vi "Lever.vi"(1 "Input":bool) -> (0 "Output":bool)   [LabVIEW 2017]
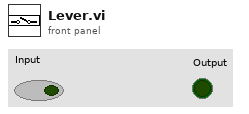
[diagram p1: front panel]
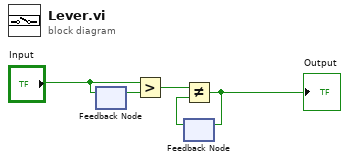
[diagram p0: block diagram]
diagram:
  n1 = feedback #1() -> (w5:bool)  [unwired: 1 in]
  n2 = feedback-in #1("Input") -> ()
  n3 = Greater?(x="Input", y=w5) -> (0:w4:bool)
  n4 = feedback #2() -> (w3:bool)  [unwired: 1 in]
  n5 = Not Equal?(x=w4, y=w3) -> (x != y?=w1:bool)
  "Output" <- w1
  n6 = feedback-in #2(w1) -> ()
